vi "Right Encoder.vi"(9 "Wheel Size":dbl=4.0, 10 "Reset":bool, 11 "Enum":enum16{"Start", "Run", "End"}(ring)) -> (2 "Rate":dbl, 3 "Distance (in)":dbl)   [LabVIEW 2014]
uses:
  TypeDefs/Digital Module 1.ctl
  <vilib>/Rock Robotics/SystemInterfaces/Typedef/FPGA_TypedefDigitalModule.ctl
  <vilib>/Rock Robotics/SystemInterfaces/DIO/FPGA_DIOChannel.ctl
  <vilib>/Rock Robotics/WPI/Encoder/WPI_EncoderType.ctl
  <vilib>/Rock Robotics/WPI/Counter/WPI_CounterDigitalInputToDigitalSource.vi
panel:
  in  "Digital Module A":T1={"Module"=enum."Digital Module 1", "L Encoder A"=enum."DIO 1", "L Encoder B"=enum."DIO 2", "R Encoder A"=enum."DIO 3", "R Encoder B"=enum."DIO 4", "Compressor"=enum."DIO 5", "Shooter Limit"=enum."DIO 6", "LED 1"=enum."DIO 7", "LED 2"=enum."DIO 8", "LED 3"=enum."DIO 9", "LED 4"=enum."DIO 9", "Shooter Limit 2"=enum."DIO 11", "Unassigned"=enum."DIO 12", "Unassigned"=enum."DIO 13", "Unassigned"=enum."DIO 14"}
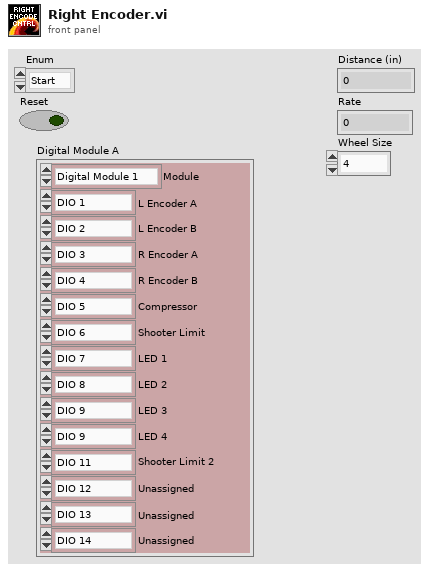
[diagram p1: front panel]
types:
  T1 = typedef "Digital Module 1.ctl" = cluster{"Module":T2, "L Encoder A":T3, "L Encoder B":T3, "R Encoder A":T3, "R Encoder B":T3, "Compressor":T3, "Shooter Limit":T3, "LED 1":T3, "LED 2":T3, "LED 3":T3, "LED 4":T3, "Shooter Limit 2":T3, "Unassigned":T3, "Unassigned":T3, "Unassigned":T3}
  T2 = typedef "FPGA_TypedefDigitalModule.ctl" = enum16{"Digital Module 1", "Digital Module 2"}
  T3 = typedef "FPGA_DIOChannel.ctl" = enum8{"DIO 1", "DIO 2", "DIO 3", "DIO 4", "DIO 5", "DIO 6", "DIO 7", "DIO 8", "DIO 9", "DIO 10", "DIO 11", "DIO 12", "DIO 13", "DIO 14", "Invalid"}
  T4 = typedef "WPI_EncoderType.ctl" = enum16{"1x", "2x", "4x"}
  T5 = typedef "WPI_DigitalInputDevRef.ctl" = cluster{"DevStatus":errorcluster, "DIO Channel":T3, "Digital Module":T2}
  T6 = typedef "FPGA_CounterEncoderSourceConvertionLVSourceType.ctl" = cluster{"DevStatus":errorcluster, "AnalogTriggerMode?":bool, "DigitalMode":cluster{"Digital Module":T2, "DIO Channel":T7}, "AnalogTriggerMode":cluster{"AnalogTriggerIndex":T8, "OutputType":T9}}
  T7 = typedef "FPGA_DIODigitalSourceChannel.ctl" = enum8{"DIO 1", "DIO 2", "DIO 3", "DIO 4", "DIO 5", "DIO 6", "DIO 7", "DIO 8", "DIO 9", "DIO 10", "DIO 11", "DIO 12", "DIO 13", "DIO 14", "Disabled"}
  T8 = typedef "FPGA_AnalogTriggerIndex.ctl" = enum8{"Trig 0", "Trig 1", "Trig 2", "Trig 3", "Trig 4", "Trig 5", "Trig 6", "Trig 7", "Invalid"}
  T9 = typedef "FPGA_AnalogTriggerOutType.ctl" = enum16{"InWindow", "TriggerState", "Rising", "Falling"}
  T10 = typedef "WPI_EncoderDevRef.ctl" = cluster{"DevStatus":errorcluster, "EncoderIndex":T11, "CounterIndex":T12, "DistancePerCount":dbl, "Decoding Type":T4}
  T11 = typedef "FPGA_EncoderIdx.ctl" = enum8{"Enc 0", "Enc 1", "Enc 2", "Enc 3", "Invalid"}
  T12 = typedef "FPGA_CounterCtrSystemIndex.ctl" = enum8{"Ctr 0", "Ctr 1", "Ctr 2", "Ctr 3", "Ctr 4", "Ctr 5", "Ctr 6", "Ctr 7", "Invalid"}
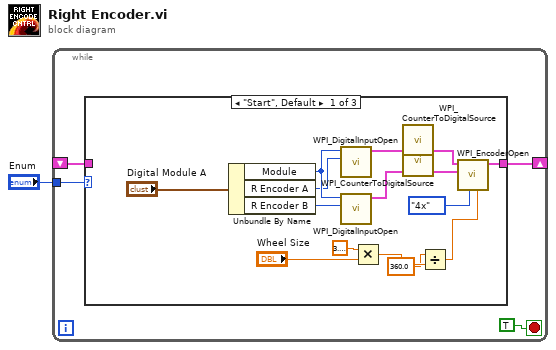
[diagram p0: block diagram]
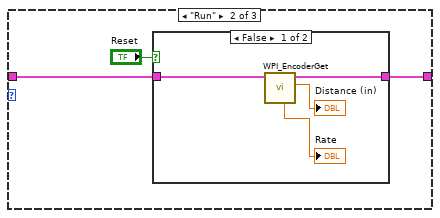
[diagram p2: hidden frame]
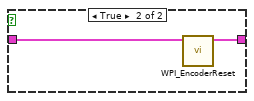
[diagram p3: hidden frame]
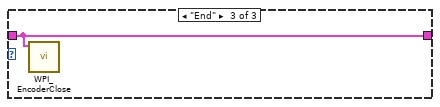
[diagram p4: hidden frame]
diagram:
  n1 = while {
    tunnel: "Enum" -> [w4]
    shift-right: [w2] -> _
    shift-left: _ -> [w3]
    stop <- TRUE stop-if-true
    n2 = case shown="\"Start\", Default" w4 {
      tunnel: w3 -> [_ w22 w30]
      tunnel: [w15 w23 w30] -> w2
      frame "Start", Default {
        n3 = Unbundle By Name("Digital Module A") -> ("Module"=w8:T2, "R Encoder A"=w7:T3, "R Encoder B"=w6:T3)
        n4 = call <vilib>:"WPI_DigitalInputOpen.vi"("DIO Channel"=w7, "Digital Module (Module 1)"=w8) -> ("DigitalInputDevRef"=w20:T5)  [unwired: 8 in, 1 out]
        n5 = call <vilib>:"WPI_DigitalInputOpen.vi"("DIO Channel"=w6, "Digital Module (Module 1)"=w8) -> ("DigitalInputDevRef"=w19:T5)  [unwired: 8 in, 1 out]
        n6 = Multiply(x=3.141592653589793, y="Wheel Size") -> (x*y=w12:dbl)
        n7 = call-poly <vilib>:"WPI_CounterToDigitalSource.vi"("DigitalInputDevRef"=w20) -> ("Digital Source"=w18:T6)  [unwired: 6 in]
        n8 = call-poly <vilib>:"WPI_CounterToDigitalSource.vi"("DigitalInputDevRef"=w19) -> ("Digital Source"=w17:T6)  [unwired: 6 in]
        n9 = Divide(x=360.0 ("y"), y=w12) -> (x/y=w10:dbl)
        n10 = call <vilib>:"WPI_EncoderOpen.vi"("DistancePerCount"=w10, "Decoding Type"=WPI_EncoderType."4x", "BSource"=w17, "ASource"=w18) -> ("EncoderDevRef"=w15:T10)  [unwired: 6 in, 1 out]
      }
      frame "Run" {
        n11 = case shown="False" "Reset" {
          tunnel: [w27 w28] -> w23
          tunnel: w22 -> [w26 w29]
          frame False {
            n12 = call <vilib>:"WPI_EncoderGet.vi"("EncoderDevRef"=w26) -> ("Distance"=→"Distance (in)":dbl, "EncoderDevRef"=w27:T10, "Rate"=→"Rate":dbl)  [unwired: 5 in, 3 out]
          }
          frame True {
            n13 = call <vilib>:"WPI_EncoderReset.vi"("EncoderDevRef"=w29) -> ("EncoderDevRef"=w28:T10)  [unwired: 9 in, 1 out]
          }
        }
      }
      frame "End" {
        n14 = call <vilib>:"WPI_EncoderClose.vi"("EncoderDevRef"=w30) -> ()  [unwired: 10 in, 1 out]
      }
    }
  }
